vi "add text to image.vi"() -> ()   [LabVIEW 2012, in "LightPipes.lvlib"]
uses:
  LightPipes.lvlib
panel:
  out "new picture":picture
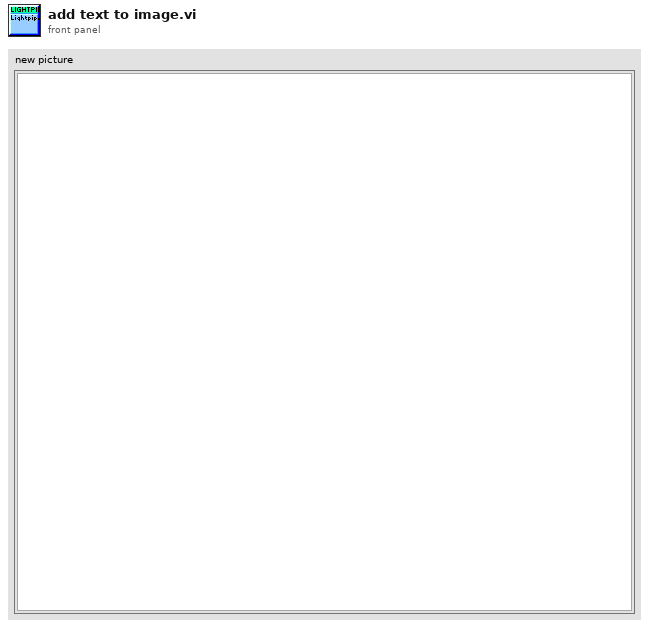
[diagram p1: front panel]
types:
  T1 = enum16{"User-specified Font", "Application Font", "System Font", "Dialog Font"}
  T2 = cluster{"horizontal":enum16{"left", "center", "right"}, "vertical":enum16{"top", "center", "bottom"}}
  T3 = typedef "imagedata.ctl" = cluster{"image type":i32, "image depth":i32, "image":u8[], "mask":u8[], "colors":u32[], "Rectangle":cluster{"left":i16, "top":i16, "right":i16, "bottom":i16}}
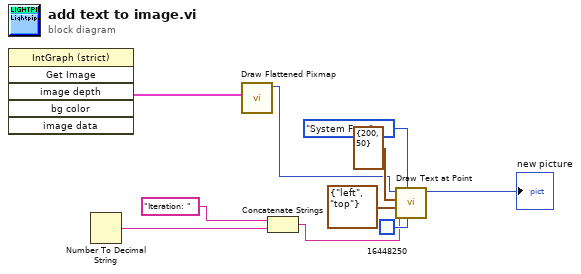
[diagram p0: block diagram]
diagram:
  n1 = invoke on="Invoke Node" class="IntGraph (strict)" method="Get Image"() -> ("image data"=w4:T3)  [unwired: 6 in, 5 out]
  n2 = Number To Decimal String() -> (decimal integer string=w2:string)  [unwired: 2 in]
  n3 = call <vilib>:"Draw Flattened Pixmap.vi"("image data"=w4) -> ("new picture"=w5:picture)  [unwired: 8 in]
  n4 = Concatenate Strings("Iteration: " ("text"), w2) -> (w1:string)
  n5 = call <vilib>:"Draw Text at Point.vi"("text color(black)"=u32 16448250, "desired font(Application)"=T1."System Font", "text"=w1, "alignment(left, top)"=T2 {"horizontal"=enum."left", "vertical"=enum."top"}, "origin"=cluster{"x":i16, "y":i16} {"x"=200, "y"=50}, "picture"=w5) -> ("new picture"=→"new picture":picture)  [unwired: 4 in, 1 out]
